vi "disable empty elements.vi"(0 "control ref":refnum<vi>, 2 "State":T1, 3 "array size":i32, 5 "error in (no error)":errorcluster) -> (19 "error out":errorcluster)   [LabVIEW 2014, in "PTScanner.lvlib" / "scan method parameters.xctl"]
uses:
  scan method parameters.xctl
  scan method parameters.State.ctl
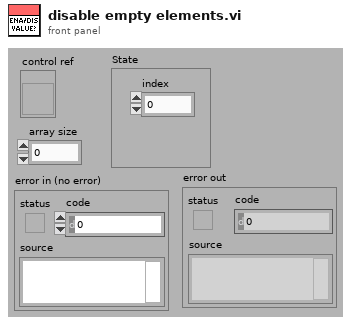
[diagram p1: front panel]
types:
  T1 = typedef "PTScanner.lvlib/scan method parameters.xctl/scan method parameters.State.ctl" = cluster{"index":i32}
  T2 = enum8{"Enabled", "Disabled", "Disabled and Grayed Out"}
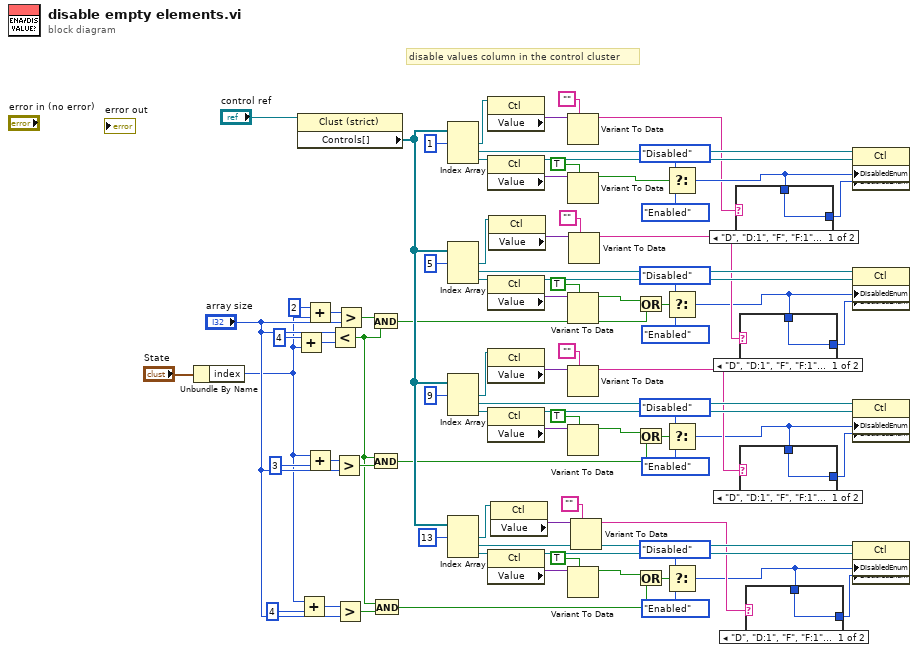
[diagram p0: block diagram]
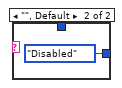
[diagram p2: hidden frame]
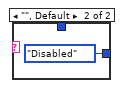
[diagram p3: hidden frame]
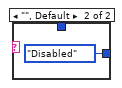
[diagram p4: hidden frame]
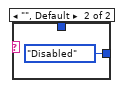
[diagram p5: hidden frame]
diagram:
  # "disable values column in the control cluster"
  n1 = Unbundle By Name("State") -> ("index"=w29:i32)
  n2 = Add(x=4, y=w29) -> (x+y=w39:i32)
  n3 = property class="Clust (strict)"(reference="control ref") -> ("Controls[]"=w83:refnum<vi>[])  [unwired: 1 in, 2 out]
  n4 = Add(x=w29, y=4) -> (x+y=w35:i32)
  n5 = Add(x=2, y=w29) -> (x+y=w38:i32)
  n6 = Add(x=w29, y=3) -> (x+y=w36:i32)
  n7 = Less?(x="array size", y=w39) -> (x < y?=w42:bool)
  n8 = Greater?(x=w36, y="array size") -> (0:w57:bool)
  n9 = Greater?(x=w35, y="array size") -> (0:w43:bool)
  n10 = Greater?(x=w38, y="array size") -> (0:w70:bool)
  n11 = And(x=w70, y=w42) -> (x .and. y?=w63:bool)
  n12 = And(x=w42, y=w57) -> (x .and. y?=w50:bool)
  n13 = And(x=w42, y=w43) -> (x .and. y?=w41:bool)
  n14 = Index Array(array=w83, index #1=1) -> (element #1=w15:refnum<vi>, element #2=w67:refnum<vi>, element #3=w81:refnum<vi>)  [unwired: 2 in]
  n15 = Index Array(array=w83, index #1=5) -> (element #1=w14:refnum<vi>, element #2=w59:refnum<vi>, element #3=w77:refnum<vi>)  [unwired: 2 in]
  n16 = Index Array(array=w83, index #1=9) -> (element #1=w24:refnum<vi>, element #2=w52:refnum<vi>, element #3=w71:refnum<vi>)  [unwired: 2 in]
  n17 = Index Array(array=w83, index #1=13) -> (element #1=w1:refnum<vi>, element #2=w45:refnum<vi>, element #3=w72:refnum<vi>)  [unwired: 2 in]
  n18 = property class="Ctl"(reference=w15) -> ("Value"=w16:variant)  [unwired: 1 in, 2 out]
  n19 = property class="Ctl"(reference=w81) -> (reference out=w66:refnum<vi>, "Value"=w82:variant)  [unwired: 1 in, 1 out]
  n20 = property class="Ctl"(reference=w77) -> (reference out=w58:refnum<vi>, "Value"=w79:variant)  [unwired: 1 in, 1 out]
  n21 = property class="Ctl"(reference=w24) -> ("Value"=w23:variant)  [unwired: 1 in, 2 out]
  n22 = property class="Ctl"(reference=w71) -> (reference out=w51:refnum<vi>, "Value"=w76:variant)  [unwired: 1 in, 1 out]
  n23 = property class="Ctl"(reference=w72) -> (reference out=w44:refnum<vi>, "Value"=w74:variant)  [unwired: 1 in, 1 out]
  n24 = property class="Ctl"(reference=w14) -> ("Value"=w19:variant)  [unwired: 1 in, 2 out]
  n25 = property class="Ctl"(reference=w1) -> ("Value"=w20:variant)  [unwired: 1 in, 2 out]
  n26 = Variant To Data(type="", Variant=w16) -> (data=w11:string)  [unwired: 1 in, 1 out]
  n27 = Variant To Data(type=TRUE, Variant=w82) -> (data=w65:bool)  [unwired: 1 in, 1 out]
  n28 = Variant To Data(type=TRUE, Variant=w79) -> (data=w64:bool)  [unwired: 1 in, 1 out]
  n29 = Variant To Data(type="", Variant=w23) -> (data=w6:string)  [unwired: 1 in, 1 out]
  n30 = Variant To Data(type=TRUE, Variant=w76) -> (data=w54:bool)  [unwired: 1 in, 1 out]
  n31 = Variant To Data(type=TRUE, Variant=w74) -> (data=w47:bool)  [unwired: 1 in, 1 out]
  n32 = Variant To Data(type="", Variant=w19) -> (data=w7:string)  [unwired: 1 in, 1 out]
  n33 = Variant To Data(type="", Variant=w20) -> (data=w5:string)  [unwired: 1 in, 1 out]
  n34 = Or(x=w64, y=w63) -> (x .or. y?=w62:bool)
  n35 = Or(x=w54, y=w50) -> (x .or. y?=w53:bool)
  n36 = Or(x=w47, y=w41) -> (x .or. y?=w46:bool)
  n37 = Select(t=T2."Disabled" ("Disabled"), s=w65, f=T2."Enabled" ("Disabled")) -> (s? t:f=w13:T2)
  n38 = Select(t=T2."Disabled" ("Disabled"), s=w62, f=T2."Enabled" ("Disabled")) -> (s? t:f=w2:T2)
  n39 = Select(t=T2."Disabled" ("Disabled"), s=w53, f=T2."Enabled" ("Disabled")) -> (s? t:f=w3:T2)
  n40 = Select(t=T2."Disabled" ("Disabled"), s=w46, f=T2."Enabled" ("Disabled")) -> (s? t:f=w4:T2)
  n41 = case shown="\"D\", \"D:1\", \"F\", \"F:1\", \"I\", \"I:1\", \"L\", \"L:1\"" w11 {
    tunnel: [w84 T2."Disabled" ("Disabled")] -> w12
    tunnel: w13 -> [w84 _]
    frame "D", "D:1", "F", "F:1", "I", "I:1", "L", "L:1" {
    }
    frame "", Default {
    }
  }
  n42 = case shown="\"D\", \"D:1\", \"F\", \"F:1\", \"I\", \"I:1\", \"L\", \"L:1\"" w7 {
    tunnel: [w86 T2."Disabled" ("Disabled")] -> w8
    tunnel: w2 -> [w86 _]
    frame "D", "D:1", "F", "F:1", "I", "I:1", "L", "L:1" {
    }
    frame "", Default {
    }
  }
  n43 = case shown="\"D\", \"D:1\", \"F\", \"F:1\", \"I\", \"I:1\", \"L\", \"L:1\"" w6 {
    tunnel: [w88 T2."Disabled" ("Disabled")] -> w10
    tunnel: w3 -> [w88 _]
    frame "D", "D:1", "F", "F:1", "I", "I:1", "L", "L:1" {
    }
    frame "", Default {
    }
  }
  n44 = case shown="\"D\", \"D:1\", \"F\", \"F:1\", \"I\", \"I:1\", \"L\", \"L:1\"" w5 {
    tunnel: [w90 T2."Disabled" ("Disabled")] -> w9
    tunnel: w4 -> [w90 _]
    frame "D", "D:1", "F", "F:1", "I", "I:1", "L", "L:1" {
    }
    frame "", Default {
    }
  }
  n45 = property class="Ctl"(reference=w67, "DisabledEnum"=w13) -> ()  [unwired: 1 in, 2 out]
  n46 = property class="Ctl"(reference=w66, "DisabledEnum"=w12) -> ()  [unwired: 1 in, 2 out]
  n47 = property class="Ctl"(reference=w59, "DisabledEnum"=w2) -> ()  [unwired: 1 in, 2 out]
  n48 = property class="Ctl"(reference=w58, "DisabledEnum"=w8) -> ()  [unwired: 1 in, 2 out]
  n49 = property class="Ctl"(reference=w52, "DisabledEnum"=w3) -> ()  [unwired: 1 in, 2 out]
  n50 = property class="Ctl"(reference=w51, "DisabledEnum"=w10) -> ()  [unwired: 1 in, 2 out]
  n51 = property class="Ctl"(reference=w45, "DisabledEnum"=w4) -> ()  [unwired: 1 in, 2 out]
  n52 = property class="Ctl"(reference=w44, "DisabledEnum"=w9) -> ()  [unwired: 1 in, 2 out]
